vi "setOutputWaveform.vi"(7 "Channel":string="0", 8 "error in (no error)":errorcluster, 10 "Type":T1, 11 "FgenKeysight in":refnum<class "ArbKeysight.lvclass">) -> (0 "error out":errorcluster, 3 "FgenKeysight out":refnum<class "ArbKeysight.lvclass">)   [LabVIEW 2023, in "ArbKeysight.lvclass"]
doc: "<b>Author:</b> Wolfgang\n<b>Description:</b> Set waveform type per channel"
uses:
  ArbKeysight.lvclass
  Data/arbWaveformType.ctl
  ArbKeysight.lvclass/ArbKeysight.ctl
  Arb.lvclass
  Driver/Keysight-33500B.lvlib
  sweArb.lvlib
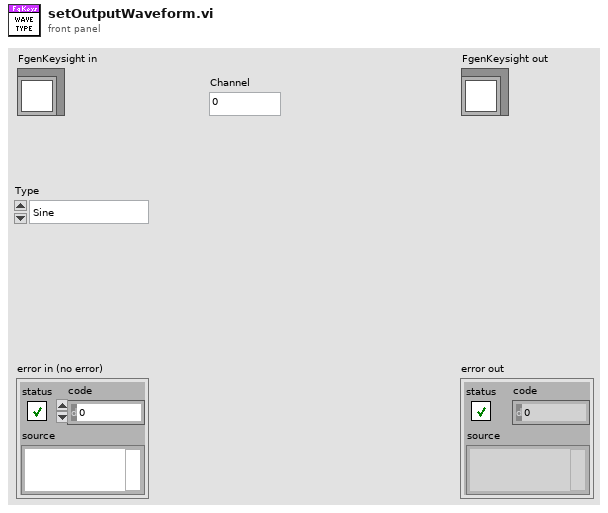
[diagram p1: front panel]
types:
  T1 = typedef "sweArb.lvlib/arbWaveformType.ctl" = enum16{"Sine", "Square", "Triangle", "DC", "Noise", "Arb"}
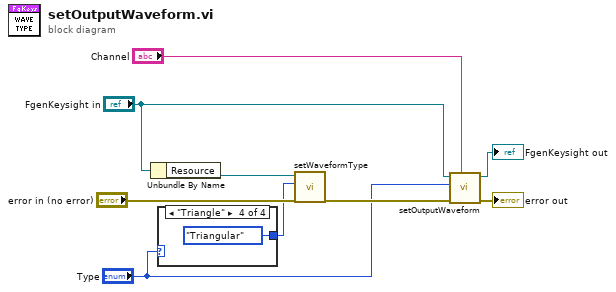
[diagram p0: block diagram]
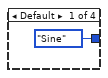
[diagram p2: hidden frame]
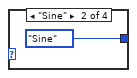
[diagram p3: hidden frame]
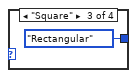
[diagram p4: hidden frame]
diagram:
  n1 = Unbundle By Name("FgenKeysight in") -> ("Resource"=w5:refnum<visa-resource-name>)
  n2 = case shown="\"Triangle\"" "Type" {
    tunnel: [enum16{"Sine", "Rectangular", "Triangular"}."Sine" ("Waveform") enum16{"Sine", "Rectangular", "Triangular"}."Sine" ("Waveform") enum16{"Sine", "Rectangular", "Triangular"}."Rectangular" ("Waveform") enum16{"Sine", "Rectangular", "Triangular"}."Triangular" ("Waveform")] -> w1
    frame Default {
    }
    frame "Sine" {
    }
    frame "Square" {
    }
    frame "Triangle" {
    }
  }
  n3 = call "setWaveformType.vi"("error in (no error)"="error in (no error)", "Waveform"=w1, "VISA resource name"=w5) -> ("error out"=w3:errorcluster)  [unwired: 7 in, 1 out]
  n4 = call-parent "setOutputWaveform.vi"("Channel"="Channel", "error in (no error)"=w3, "Type"="Type", "Fgen in"="FgenKeysight in") -> ("error out"=→"error out":errorcluster, "Fgen out"=→"FgenKeysight out":refnum<class "ArbKeysight.lvclass">)  [unwired: 6 in]
